vi "Update Current Execution Time.vi"(8 "error in":errorcluster, 10 "Current Execution Time (us)":u32, 11 "Execution Unit in":refnum<class "Execution Unit.lvclass">) -> (0 "error out":errorcluster, 3 "Execution Unit out":refnum<class "Execution Unit.lvclass">)   [LabVIEW 2023, in "Ballard MIL-STD-1553 Engine Support.lvlib" / "Implementation.lvlib" / "Execution Unit.lvclass"]
uses:
  Execution Unit.lvclass
  Execution Unit.lvclass/Execution Unit.ctl
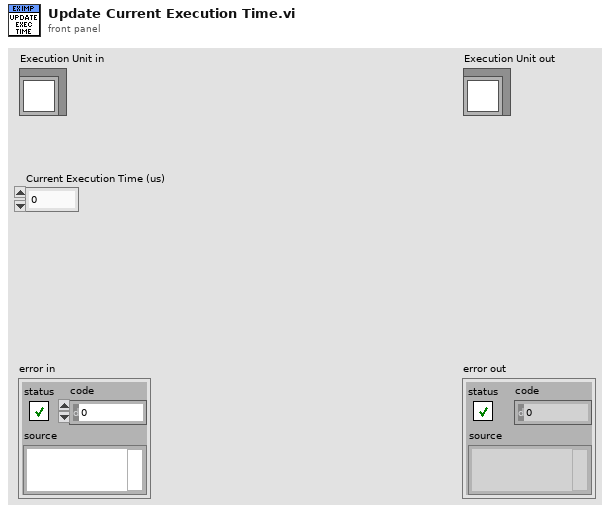
[diagram p1: front panel]
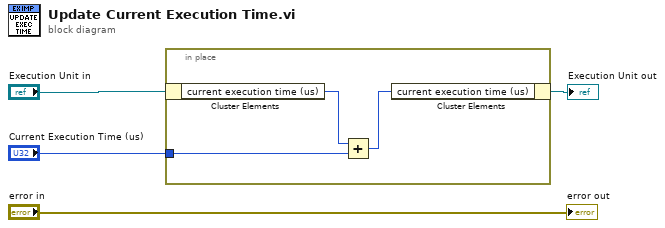
[diagram p0: block diagram]
diagram:
  n1 = in-place {
    in-place-border: "Current Execution Time (us)" -> [w7]
    n2 = in-place-cluster #1("Execution Unit in") -> ("current execution time (us)"=w6:u32)
    n3 = Add(x=w6, y=w7) -> (x+y=w5:u32)
    n4 = in-place-cluster #1("current execution time (us)"=w5) -> (→"Execution Unit out":refnum<class "Execution Unit.lvclass">)
  }
  "error out" <- "error in"
